vi "Button Read.vi"(8 "error in (no error)":errorcluster, 11 "HG_LIB in":T1) -> (0 "error out":errorcluster, 1 "Stop":bool, 2 "Start":bool, 3 "HG_LIB out":T2)   [LabVIEW 2020]
uses:
  <vilib>/High Genius/HG_WSI_Tookit/Dependencies/Library/Digital Input and Output/Digital Input and Output.lvclass
  C:/Program Files (x86)/National Instruments/LabVIEW 2020/vi.lib/High Genius/HG_WSI_Tookit/Dependencies/Library/HG_LIB/HG_LIB.lvclass
  <vilib>/High Genius/HG_WSI_Tookit/Dependencies/Library/HG_LIB/HG_LIB.lvclass/HG_LIB.ctl
  <vilib>/High Genius/HG_WSI_Tookit/Dependencies/Library/HG_LIB/HG_LIB.lvclass
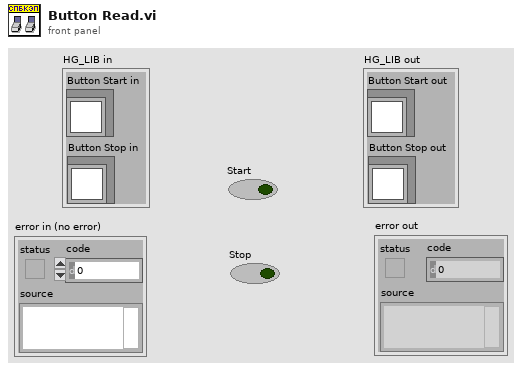
[diagram p1: front panel]
types:
  T1 = cluster{"Button Start in":refnum<class "Digital Input and Output.lvclass">, "Button Stop in":refnum<class "Digital Input and Output.lvclass">}
  T2 = cluster{"Button Start out":refnum<class "Digital Input and Output.lvclass">, "Button Stop out":refnum<class "Digital Input and Output.lvclass">}
  T3 = cluster{"data":cluster{"ai22":sgl, "ai23":sgl, "ai24":sgl, "ai25":sgl, "pulse12":i32, "pulse13":i32, "pwm14":i32, "pwm15":i32, "pwm16":i32, "do17":bool, "do18":bool, "do19":bool, "do20":bool, "do21":bool, "di11":bool, "di9":bool, "motor0":u8, "motor1":u8, "motor2":u8, "motor3":u8, "dir00":u8, "dir01":u8, "dir02":u8, "dir03":u8, "dir10":u8, "dir11":u8, "dir12":u8, "dir13":u8, "limit0":bool, "limit1":bool, "limit2":bool, "limit3":bool, "limit4":bool, "limit5":bool, "limit6":bool, "limit7":bool, "lsb0H":u8, "lsb1H":u8, "lsb2H":u8, "lsb3H":u8, "lsb0L":u8, "lsb1L":u8, "lsb2L":u8, "lsb3L":u8, "enc0_counters":u32, "enc1_counters":u32, "enc2_counters":u32, "enc3_counters":u32, "counter10":u32, "counter8":u32, "reset_enc0":bool, "reset_enc1":bool, "reset_enc2":bool, "reset_enc3":bool, "pitch":sgl, "roll":sgl, "yaw":sgl, "zero_yaw":bool}}
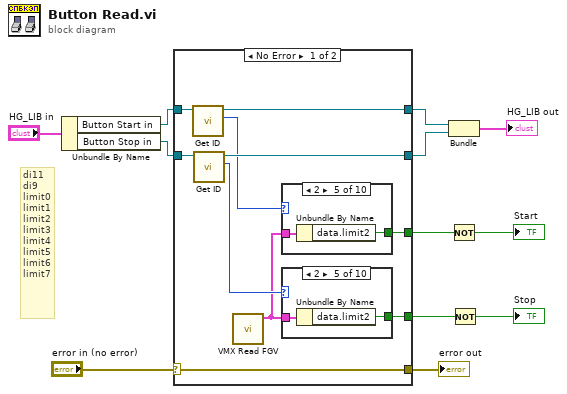
[diagram p0: block diagram]
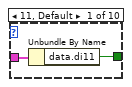
[diagram p2: hidden frame]
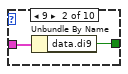
[diagram p3: hidden frame]
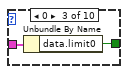
[diagram p4: hidden frame]
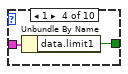
[diagram p5: hidden frame]
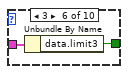
[diagram p6: hidden frame]
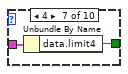
[diagram p7: hidden frame]
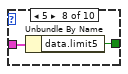
[diagram p8: hidden frame]
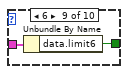
[diagram p9: hidden frame]
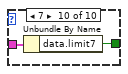
[diagram p10: hidden frame]
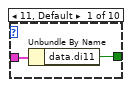
[diagram p11: hidden frame]
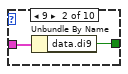
[diagram p12: hidden frame]
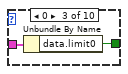
[diagram p13: hidden frame]
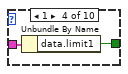
[diagram p14: hidden frame]
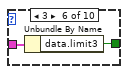
[diagram p15: hidden frame]
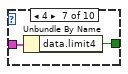
[diagram p16: hidden frame]
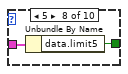
[diagram p17: hidden frame]
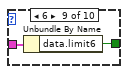
[diagram p18: hidden frame]
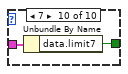
[diagram p19: hidden frame]
diagram:
  # "di11\ndi9\nlimit0\nlimit1\nlimit2\nlimit3\nlimit4\nlimit5\nlimit6\nlimit7"
  n1 = Unbundle By Name("HG_LIB in") -> ("Button Start in"=w2:refnum<class "Digital Input and Output.lvclass">, "Button Stop in"=w1:refnum<class "Digital Input and Output.lvclass">)
  n2 = case shown="No Error" "error in (no error)" {
    selector: "error in (no error)" -> [w18 w65]
    tunnel: [w18 w65] -> w11
    tunnel: [w21 w64] -> w9
    tunnel: w1 -> [w22 w64]
    tunnel: [w19 _] -> w6
    tunnel: w2 -> [w17 w63]
    tunnel: [w15 w63] -> w10
    tunnel: [w13 _] -> w7
    frame No Error {
      n3 = call <vilib>:"Get ID.vi"("HG_LIB in"=w17) -> ("ID"=w16:u32, "HG_LIB out"=w15:refnum<class "Digital Input and Output.lvclass">)  [unwired: 9 in]
      n4 = call <vilib>:"Get ID.vi"("HG_LIB in"=w22) -> ("ID"=w20:u32, "HG_LIB out"=w21:refnum<class "Digital Input and Output.lvclass">)  [unwired: 9 in]
      n5 = call <vilib>:"VMX Read FGV.vi"() -> ("Read Data"=w14:T3)  [unwired: 10 in, 1 out]
      n6 = case shown="2" w16 {
        tunnel: w14 -> [w24 w26 w27 w30 w31 w34 w36 w38 w40 w42]
        tunnel: [w23 w25 w28 w29 w32 w33 w35 w37 w39 w41] -> w13
        frame 11, Default {
          n7 = Unbundle By Name(w24) -> ("data.di11"=w23:bool)
        }
        frame 9 {
          n8 = Unbundle By Name(w26) -> ("data.di9"=w25:bool)
        }
        frame 0 {
          n9 = Unbundle By Name(w27) -> ("data.limit0"=w28:bool)
        }
        frame 1 {
          n10 = Unbundle By Name(w30) -> ("data.limit1"=w29:bool)
        }
        frame 2 {
          n11 = Unbundle By Name(w31) -> ("data.limit2"=w32:bool)
        }
        frame 3 {
          n12 = Unbundle By Name(w34) -> ("data.limit3"=w33:bool)
        }
        frame 4 {
          n13 = Unbundle By Name(w36) -> ("data.limit4"=w35:bool)
        }
        frame 5 {
          n14 = Unbundle By Name(w38) -> ("data.limit5"=w37:bool)
        }
        frame 6 {
          n15 = Unbundle By Name(w40) -> ("data.limit6"=w39:bool)
        }
        frame 7 {
          n16 = Unbundle By Name(w42) -> ("data.limit7"=w41:bool)
        }
      }
      n17 = case shown="2" w20 {
        tunnel: w14 -> [w44 w46 w47 w50 w51 w54 w56 w58 w60 w62]
        tunnel: [w43 w45 w48 w49 w52 w53 w55 w57 w59 w61] -> w19
        frame 11, Default {
          n18 = Unbundle By Name(w44) -> ("data.di11"=w43:bool)
        }
        frame 9 {
          n19 = Unbundle By Name(w46) -> ("data.di9"=w45:bool)
        }
        frame 0 {
          n20 = Unbundle By Name(w47) -> ("data.limit0"=w48:bool)
        }
        frame 1 {
          n21 = Unbundle By Name(w50) -> ("data.limit1"=w49:bool)
        }
        frame 2 {
          n22 = Unbundle By Name(w51) -> ("data.limit2"=w52:bool)
        }
        frame 3 {
          n23 = Unbundle By Name(w54) -> ("data.limit3"=w53:bool)
        }
        frame 4 {
          n24 = Unbundle By Name(w56) -> ("data.limit4"=w55:bool)
        }
        frame 5 {
          n25 = Unbundle By Name(w58) -> ("data.limit5"=w57:bool)
        }
        frame 6 {
          n26 = Unbundle By Name(w60) -> ("data.limit6"=w59:bool)
        }
        frame 7 {
          n27 = Unbundle By Name(w62) -> ("data.limit7"=w61:bool)
        }
      }
    }
    frame Error {
    }
  }
  "error out" <- w11
  n28 = Bundle("Button Start in"=w10, "Button Stop in"=w9) -> (→"HG_LIB out":T1)  [unwired: 1 in]
  n29 = Not(x=w7) -> (.not. x?=→"Start":bool)
  n30 = Not(x=w6) -> (.not. x?=→"Stop":bool)
